vi "blue_freq_off_first.vi"(8 "error in (no error)":errorcluster, 10 "LED CONTROLS":dbl[][](array[numeric]), 11 "Iteration in":u32) -> (0 "error out":errorcluster, 3 "Iteration out":u32)   [LabVIEW 2013]
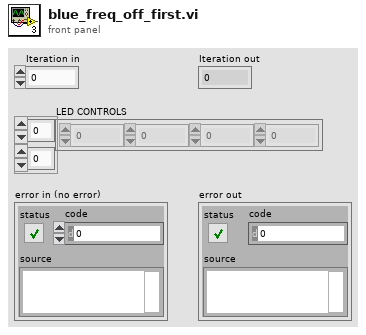
[diagram p1: front panel]
types:
  T1 = enum16{"Set Mode", "Set Normal Current ", "Set Strobe Parameters", "Set Normal Parameters", "Set Strobe Profile "}
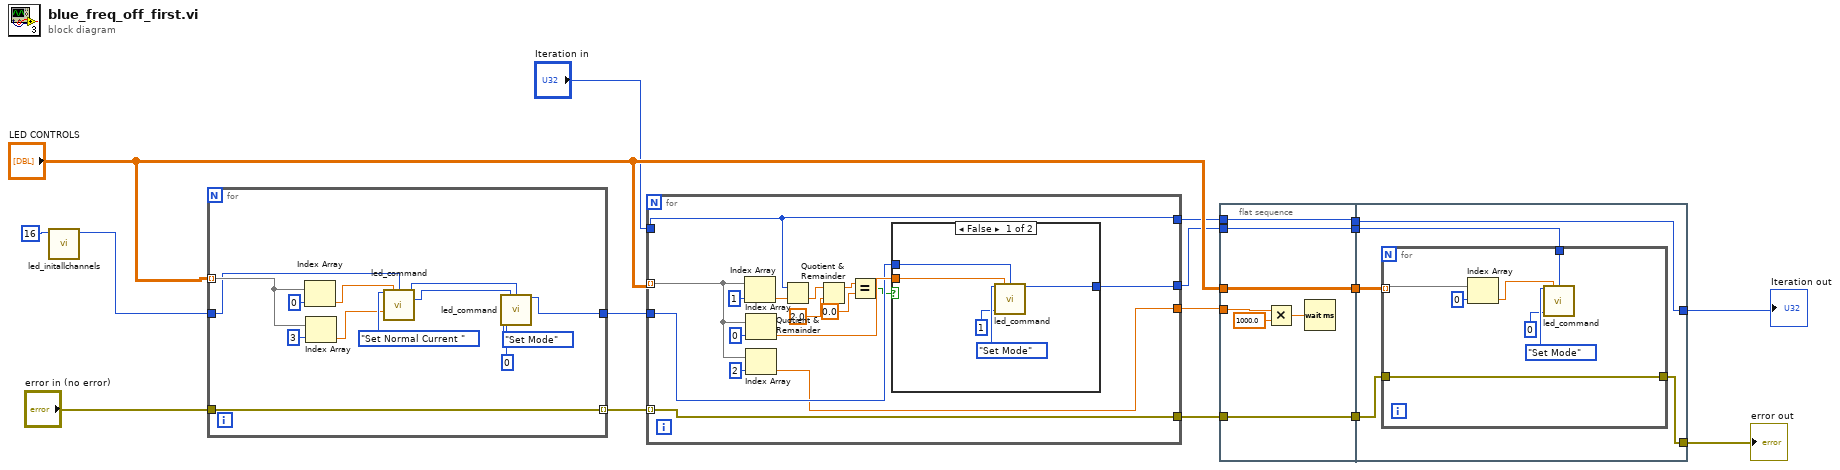
[diagram p0: block diagram]
diagram:
  n1 = call "led_initallchannels.vi"("Channels"=16) -> ("Device Handle Out"=w1:u32)  [unwired: 9 in, 1 out]
  n2 = for {
    tunnel: "error in (no error)" -> [w30]
    tunnel: [w30] -> w11 mode=indexing
    tunnel: w1 -> [w19]
    tunnel: [w18] -> w12
    tunnel: "LED CONTROLS" -> [w20] mode=indexing
    n3 = Index Array(array=w20, index=0) -> (element=w27:dbl)
    n4 = Index Array(array=w20, index=3) -> (element=w25:dbl)
    n5 = call "led_command.vi"("COMMAND"=T1."Set Normal Current ", "Channel"=w27, "Device Handle"=w19, "Iset"=w25) -> ("Device Handle Out"=w22:u32, "Channel Out"=w23:i32)  [unwired: 8 in, 2 out]
    n6 = call "led_command.vi"("COMMAND"=T1."Set Mode", "Channel"=w23, "Device Handle"=w22, "Mode"=u32 0) -> ("Device Handle Out"=w18:u32)  [unwired: 8 in, 3 out]
  }
  n7 = for {
    tunnel: "Iteration in" -> [w38]
    tunnel: "LED CONTROLS" -> [w36] mode=indexing
    tunnel: w12 -> [w41]
    tunnel: [w40] -> w4
    tunnel: [w39] -> w5
    tunnel: [w38] -> w6
    tunnel: [w37] -> w8
    tunnel: w11 -> [w37] mode=indexing
    n8 = Index Array(array=w36, index=1) -> (element=w45:dbl)
    n9 = Index Array(array=w36, index=0) -> (element=w42:dbl)
    n10 = Index Array(array=w36, index=2) -> (element=w40:dbl)
    n11 = Quotient & Remainder(x=w38, y=w45) -> (floor(x/y)=w35:dbl)  [unwired: 1 out]
    n12 = Quotient & Remainder(x=w35, y=2.0) -> (x-y*floor(x/y)=w33:dbl)  [unwired: 1 out]
    n13 = Equal?(x=w33, y=0.0) -> (x = y?=w31:bool)
    n14 = case shown="False" w31 {
      tunnel: w42 -> [w49 _]
      tunnel: w41 -> [w48 w52]
      tunnel: [w47 w52] -> w39
      frame False {
        n15 = call "led_command.vi"("COMMAND"=T1."Set Mode", "Channel"=w49, "Device Handle"=w48, "Mode"=u32 1) -> ("Device Handle Out"=w47:u32)  [unwired: 8 in, 3 out]
      }
      frame True {
      }
    }
  }
  n16 = flat-sequence {
    tunnel: "LED CONTROLS" -> [w59]
    tunnel: w4 -> [w58]
    tunnel: [w59] -> w17
    tunnel: w5 -> [w55]
    tunnel: [w55] -> w16
    tunnel: w6 -> [w54]
    tunnel: [w54] -> w15
    tunnel: w8 -> [w53]
    tunnel: [w53] -> w14
    tunnel: w17 -> [w64]
    tunnel: w16 -> [w63]
    tunnel: w15 -> [w62]
    tunnel: [w62] -> w7
    tunnel: w14 -> [w61]
    tunnel: [w60] -> w9
    frame #0 {
      n17 = Multiply(x=w58, y=1000.0) -> (x*y=w57:dbl)
      n18 = Wait (ms)(milliseconds to wait=w57) -> ()  [unwired: 1 out]
    }
    frame #1 {
      n19 = for {
        tunnel: w64 -> [w65] mode=indexing
        tunnel: w63 -> [w68]
        tunnel: w61 -> [w66]
        tunnel: [w66] -> w60
        n20 = Index Array(array=w65, index=0) -> (element=w67:dbl)
        n21 = call "led_command.vi"("COMMAND"=T1."Set Mode", "Channel"=w67, "Device Handle"=w68, "Mode"=u32 0) -> ()  [unwired: 8 in, 4 out]
      }
    }
  }
  "error out" <- w9
  "Iteration out" <- w7
